vi "5650 init.vi"() -> ()   [LabVIEW 2019]
panel:
  out "measurement data":dbl[](array[numeric]) format="%#_7p"
  out "status":dbl
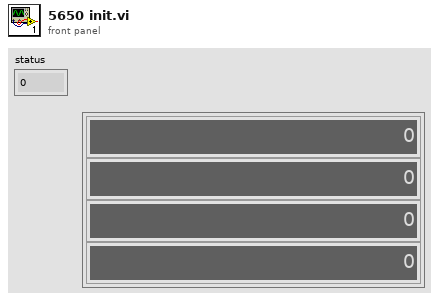
[diagram p1: front panel]
types:
  T1 = enum16{"IMAGinary", "PHASe", "REAL2", "MLINear2", "IMAGinary2", "PHASe2"}
  T2 = enum16{"REAL", "MLINear", "IMAGinary", "PHASe", "REAL2", "MLINear2"}
  T3 = enum16{"IMAGinary", "PHASe", "AUX1", "AUX2", "REAL2", "MLINear2", "IMAGinary2", "PHASe2"}
  T4 = enum16{"REAL", "MLINear", "IMAGinary", "PHASe", "NOISe", "AUX1", "REAL2", "MLINear2"}
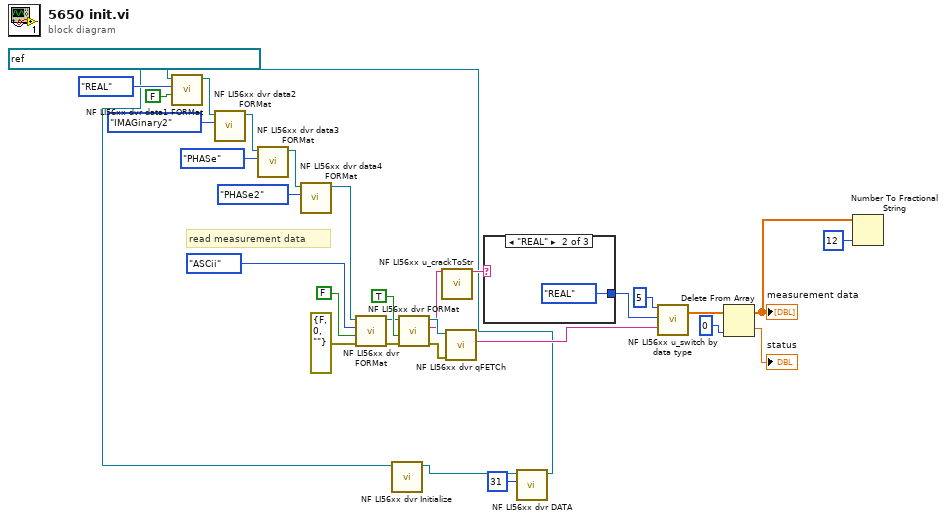
[diagram p0: block diagram]
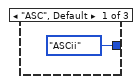
[diagram p2: hidden frame]
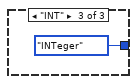
[diagram p3: hidden frame]
diagram:
  # "read measurement data"
  n1 = call "NF LI56xx dvr Initialize.vi"("VISA resource name"=refnum<visa-resource-name> "USB0::0x0D4A::0x004F::9253259::INSTR") -> ("VISA resource name out"=w6:refnum<visa-resource-name>)  [unwired: 8 in, 2 out]
  n2 = call "NF LI56xx dvr DATA.vi"("set measurement data"=u8 31, "VISA resource name"=w6) -> ("VISA resource name copy"=w3:refnum<visa-resource-name>)  [unwired: 7 in, 2 out]
  n3 = call "NF LI56xx dvr data1 FORMat.vi"("Read(F)"=FALSE, "set measurement \nparameters format"=T4."REAL" ("set measurement \nparameters format"), "VISA resource name"=w3) -> ("VISA resource name copy"=w29:refnum<visa-resource-name>)  [unwired: 6 in, 2 out]
  n4 = call "NF LI56xx dvr data2 FORMat.vi"("set measurement \nparameters format"=T3."IMAGinary2" ("set measurement \nparameters format"), "VISA resource name"=w29) -> ("VISA resource name copy"=w27:refnum<visa-resource-name>)  [unwired: 7 in, 2 out]
  n5 = call "NF LI56xx dvr data3 FORMat.vi"("set measurement \nparameters format"=T2."PHASe" ("set measurement \nparameters format"), "VISA resource name"=w27) -> ("VISA resource name copy"=w26:refnum<visa-resource-name>)  [unwired: 7 in, 2 out]
  n6 = call "NF LI56xx dvr data4 FORMat.vi"("set measurement \nparameters format"=T1."PHASe2" ("set measurement \nparameters format"), "VISA resource name"=w26) -> ("VISA resource name copy"=w23:refnum<visa-resource-name>)  [unwired: 7 in, 2 out]
  n7 = call "NF LI56xx dvr FORMat.vi"("error in"=errorcluster {"status"=FALSE, "code"=0, "source"=""} ("error out"), "Read(F)"=FALSE, "set data transfer format"=enum16{"ASCii", "REAL", "INTeger"}."ASCii", "VISA resource name"=w23) -> ("error out"=w10:errorcluster, "VISA resource name copy"=w9:refnum<visa-resource-name>)  [unwired: 5 in, 1 out]
  n8 = call "NF LI56xx dvr FORMat.vi"("error in"=w10, "Read(F)"=TRUE, "VISA resource name"=w9) -> ("error out"=w16:errorcluster, "query data transfer format"=w11:string, "VISA resource name copy"=w15:refnum<visa-resource-name>)  [unwired: 6 in]
  n9 = call "NF LI56xx u_crackToStr.vi"("input string"=w11) -> ("output string"=w12:string)  [unwired: 18 in]
  n10 = call "NF LI56xx dvr qFETCh.vi"("error in"=w16, "VISA resource name"=w15) -> ("measurement data"=w19:string)  [unwired: 7 in, 2 out]
  n11 = case shown="\"REAL\"" w12 {
    tunnel: [enum16{"ASCii", "REAL", "INTeger"}."ASCii" enum16{"ASCii", "REAL", "INTeger"}."REAL" enum16{"ASCii", "REAL", "INTeger"}."INTeger"] -> w13
    frame "ASC", Default {
    }
    frame "REAL" {
    }
    frame "INT" {
    }
  }
  n12 = call "NF LI56xx u_switch by data type.vi"("Num"=u8 5 ("数値"), "data format"=w13, "input string"=w19) -> ("query measurement data"=w18:dbl[])  [unwired: 16 in]
  n13 = Delete From Array(array=w18, index=0 ("指標")) -> (deleted portion=→"status":dbl, array with subset deleted=w2:dbl[])  [unwired: 1 in]
  "measurement data" <- w2
  n14 = Number To Fractional String(number=w2, precision (6)=i16 12) -> ()  [unwired: 2 in, 1 out]
